vi "Strip EthernetFrame (MAC).vi"(11 "Ethernet Frame In":u8[](array[numeric]) format="%.0x") -> (2 "Ethernet header":T1 {"EtherType" format="%04x"; "Src MAC" format="%02x"; "Dest MAC" format="%02x"}, 3 "Ethernet Frame Out":u8[](array[numeric]) format="%.0x")   [LabVIEW 2020, in "EthFrameManagement.lvlib"]
uses:
  EthFrameManagement.lvlib
  controls/ehternetFrame_type.ctl
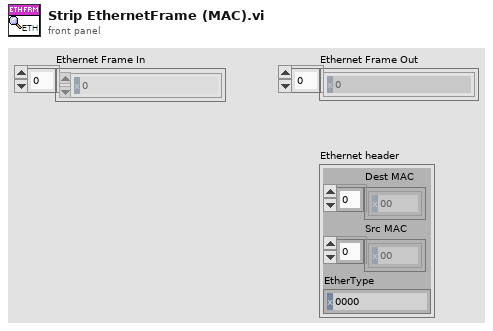
[diagram p1: front panel]
types:
  T1 = typedef "EthFrameManagement.lvlib/ehternetFrame_type.ctl" = cluster{"Dest MAC":u8[], "Src MAC":u8[], "EtherType":u16}
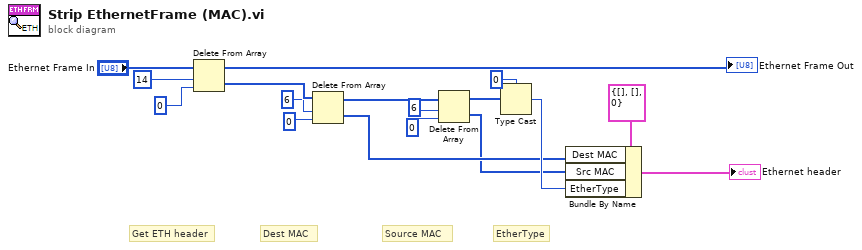
[diagram p0: block diagram]
diagram:
  # "EtherType"
  # "Get ETH header"
  # "Source MAC"
  # "Dest MAC"
  n1 = Delete From Array(array="Ethernet Frame In", length=14, index=0) -> (deleted portion=w12:u8[], array with subset deleted=→"Ethernet Frame Out":u8[])
  n2 = Delete From Array(array=w12, length=6, index=0) -> (deleted portion=w3:u8[], array with subset deleted=w11:u8[])
  n3 = Delete From Array(array=w11, length=6, index=0) -> (deleted portion=w2:u8[], array with subset deleted=w6:u8[])
  n4 = Type Cast(type=u16 0, x=w6) -> (*(type *) &x=w4:u16)
  n5 = Bundle By Name(cluster=T1 {"Dest MAC"=[], "Src MAC"=[], "EtherType"=0}, "Dest MAC"=w3, "Src MAC"=w2, "EtherType"=w4) -> (→"Ethernet header":T1)
